vi "mlog1.vi"(5 "string2":string, 6 "string1":string, 7 "message":refnum<vi>) -> ()   [LabVIEW 2010]
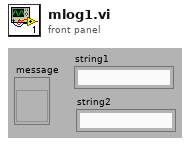
[diagram p1: front panel]
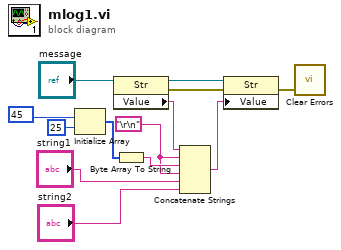
[diagram p0: block diagram]
diagram:
  w1 = "\r\n"
  n1 = Initialize Array(u8 45, 25 ("dimension size")) -> (w2:u8[])
  n2 = property class="Str"(reference="message") -> (reference out=w9:refnum<vi>, error out=w10:errorcluster, "Value"=w12:string)  [unwired: 1 in]
  n3 = Byte Array To String(unsigned byte array=w2) -> (string=w6:string)
  n4 = Concatenate Strings(w12, w1, w6, w1, "string1", "string2") -> (w13:string)
  n5 = property class="Str"(reference=w9, error in=w10, "Value"=w13) -> (error out=w11:errorcluster)  [unwired: 1 out]
  n6 = call <vilib>:"Clear Errors.vi"("error in (no error)"=w11) -> ()  [unwired: 6 in, 1 out]
